vi "Get Decendants.vi"(8 "error in (no error)":errorcluster, 11 "TargetRef in":refnum<vi>) -> (0 "error out":errorcluster, 1 "Names":string[](array[string]), 2 "Decendant References":refnum<vi>[](array[refnum]), 3 "TargetRef Out":refnum<vi>)   [LabVIEW 2015, in "Generic Module Library.lvlib"]
uses:
  Generic Module Library.lvlib
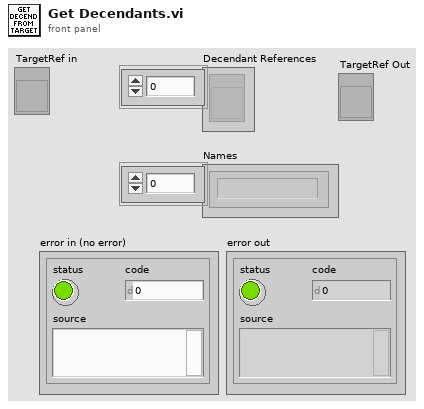
[diagram p1: front panel]
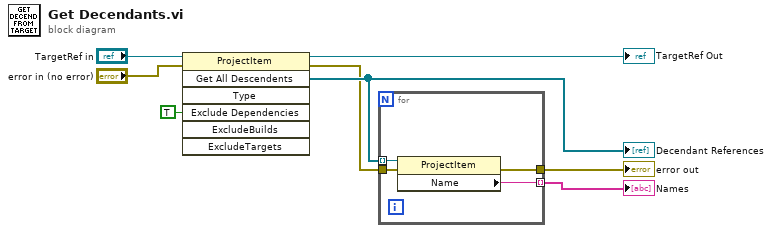
[diagram p0: block diagram]
diagram:
  n1 = invoke class="ProjectItem" method="Get All Descendents"(reference="TargetRef in", error in="error in (no error)", "Exclude Dependencies"=TRUE ("ExcludeDependencies")) -> (reference out=→"TargetRef Out":refnum<vi>, error out=w2:errorcluster, "All Descendents"=w7:refnum<vi>[])  [unwired: 4 in, 4 out]
  "Decendant References" <- w7
  n2 = for {
    tunnel: w7 -> [w12] mode=indexing
    tunnel: [w11] -> w6 mode=indexing
    tunnel: w2 -> [w10]
    tunnel: [w9] -> w1
    n3 = property class="ProjectItem"(reference=w12, error in=w10) -> (error out=w9:errorcluster, "Name"=w11:string)  [unwired: 1 out]
  }
  "Names" <- w6
  "error out" <- w1
